vi "waitForNewWaveforms.vi"(8 "error in (no error)":errorcluster, 11 "Instrument.Lockin in":refnum<class "Instrument.Lockin.lvclass">) -> (0 "error out":errorcluster, 2 "Newest AI Waveform":waveform(dbl)[](array[waveform]), 3 "Instrument.Lockin out":refnum<class "Instrument.Lockin.lvclass">)   [LabVIEW 2016, in "Instrument.Lockin.lvclass"]
uses:
  Instrument.Lockin.lvclass
  <vilib>/Utility/error.llb/Error Cluster From Error Code.vi
  <vilib>/ErrorRing/Error Ring.xnode
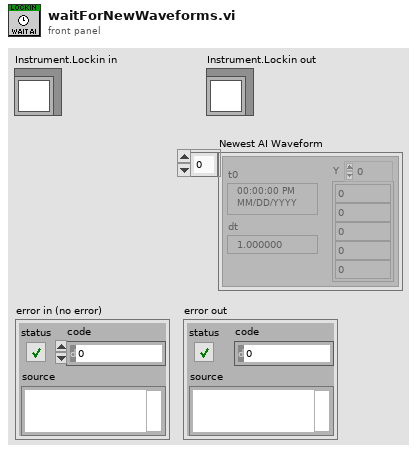
[diagram p1: front panel]
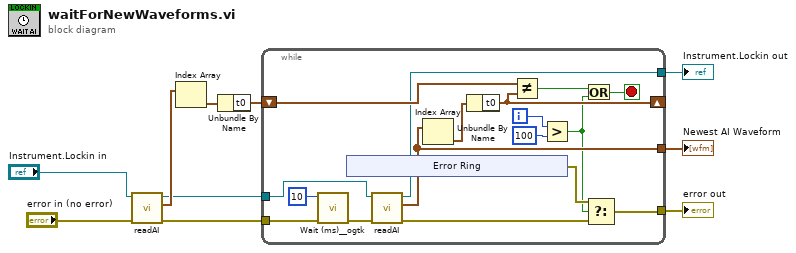
[diagram p0: block diagram]
diagram:
  n1 = call "readAI.vi"("error in (no error)"="error in (no error)", "Instrument.Lockin in"="Instrument.Lockin in") -> ("error out"=w10:errorcluster, "AI Waveform"=w4:waveform(dbl)[], "Instrument.Lockin out"=w2:refnum<class "Instrument.Lockin.lvclass">)  [unwired: 7 in]
  n2 = Index Array(array=w4) -> (element=w8:waveform(dbl))  [unwired: 1 in]
  n3 = Unbundle By Name(w8) -> ("t0"=w9:timestamp)
  n4 = while {
    shift-right: [w24] -> _
    shift-left: w9 -> [w25]
    tunnel: w10 -> [w26]
    tunnel: [w11] -> w6
    tunnel: [w21] -> w5
    tunnel: w2 -> [w20]
    tunnel: [w19] -> w1
    i -> [w18]
    stop <- w15 stop-if-true
    n5 = call <userlib>:"Wait (ms)__ogtk.vi"("error in (no error)"=w26, "milliseconds to wait"=u32 10) -> ("error out"=w23:errorcluster)  [unwired: 8 in, 1 out]
    n6 = xnode "Error Ring"() -> ("error out"=w14:errorcluster)
    n7 = call "readAI.vi"("error in (no error)"=w23, "Instrument.Lockin in"=w20) -> ("error out"=w12:errorcluster, "AI Waveform"=w21:waveform(dbl)[], "Instrument.Lockin out"=w19:refnum<class "Instrument.Lockin.lvclass">)  [unwired: 7 in]
    n8 = Index Array(array=w21) -> (element=w27:waveform(dbl))  [unwired: 1 in]
    n9 = Unbundle By Name(w27) -> ("t0"=w24:timestamp)
    n10 = Not Equal?(x=w25, y=w24) -> (x != y?=w16:bool)
    n11 = Greater?(x=w18, y=100) -> (0:w13:bool)
    n12 = Or(x=w16, y=w13) -> (x .or. y?=w15:bool)
    n13 = Select(t=w14, s=w13, f=w12) -> (s? t:f=w11:errorcluster)
  }
  "error out" <- w6
  "Newest AI Waveform" <- w5
  "Instrument.Lockin out" <- w1
